vi "enable or disable controls.vi"(9 "don't gray out":bool, 10 "disable set":refnum<vi>[](array[refnum]), 11 "enable set":refnum<vi>[](array[refnum])) -> ()   [LabVIEW 2014, in "TEC editor node.lvclass"]
uses:
  TEC editor node.lvclass
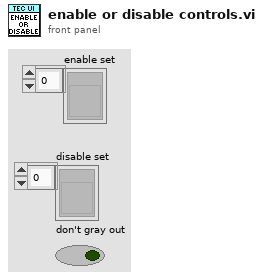
[diagram p1: front panel]
types:
  T1 = enum8{"Enabled", "Disabled", "Disabled and Grayed Out"}
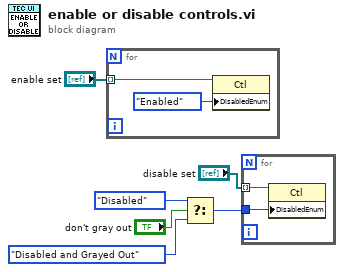
[diagram p0: block diagram]
diagram:
  n1 = for {
    tunnel: "enable set" -> [w8] mode=indexing
    n2 = property class="Ctl"(reference=w8, "DisabledEnum"=T1."Enabled" ("Disabled")) -> ()  [unwired: 1 in, 2 out]
  }
  n3 = Select(t=T1."Disabled" ("Disabled"), s="don't gray out", f=T1."Disabled and Grayed Out" ("Disabled")) -> (s? t:f=w2:T1)
  n4 = for {
    tunnel: "disable set" -> [w10] mode=indexing
    tunnel: w2 -> [w9]
    n5 = property class="Ctl"(reference=w10, "DisabledEnum"=w9) -> ()  [unwired: 1 in, 2 out]
  }
